vi "GT Get Adc Filter Prm.vi"(8 "error in (no error)":errorcluster caption="错误输入（无错误）", 9 "pk":dbl, 10 "adc":i16, 11 "cardNum":i16) -> (0 "error out":errorcluster caption="错误输出", 1 "pk out":dbl, 3 "function return":i16)   [LabVIEW 2014, in "gts.lvlib"]
doc: "GT_API GT_GetAdcFilterPrm(short cardNum,short adc,double *pk);"
uses:
  gts.lvlib
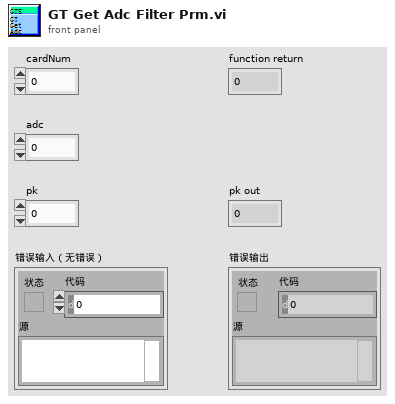
[diagram p1: front panel]
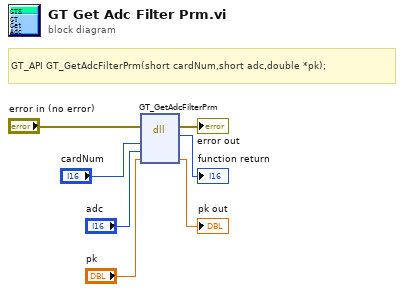
[diagram p0: block diagram]
diagram:
  # "GT_API GT_GetAdcFilterPrm(short cardNum,short adc,double *pk);"
  n1 = dll-call lib="PTH2habs D固高科技资料GTS控制卡GTS卡18年上半年资料dllVC32bit\nmulti_cardgts.*" fn="GT_GetAdcFilterPrm"(error in="error in (no error)", "cardNum"="cardNum", "adc"="adc", "pk"="pk") -> (error out=→"error out":errorcluster, →"function return":i16, "pk"=→"pk out":dbl)  [unwired: 4 in, 1 out]
